vi "From Variant.vi"(8 "error in (no error)":errorcluster, 10 "Variant":variant, 11 "Abs_Double Float in":refnum<class "Abs_U32 Integer 1D.lvclass">) -> (0 "error out":errorcluster, 3 "Abs_Double Float out":refnum<class "Abs_U32 Integer 1D.lvclass">)   [LabVIEW 2021, in "Abs_U32 Integer 1D.lvclass"]
uses:
  Abs_U32 Integer 1D.lvclass
  Support/Type.ctl
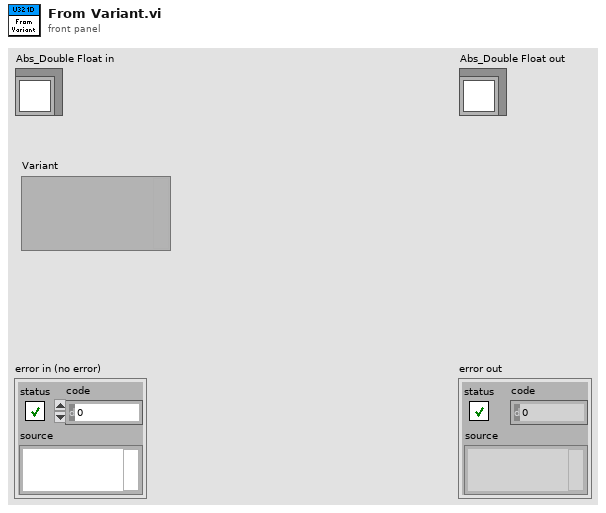
[diagram p1: front panel]
types:
  T1 = typedef "Abs_U32 Integer 1D.lvclass/Type.ctl" = u32[]
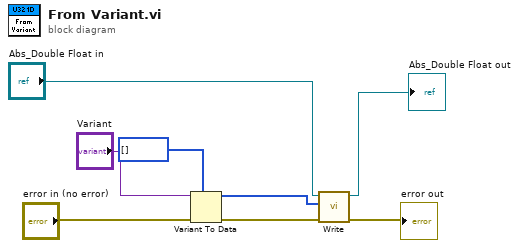
[diagram p0: block diagram]
diagram:
  n1 = Variant To Data(error in="error in (no error)", type=T1 [], Variant="Variant") -> (data=w7:T1, error out=w8:errorcluster)
  n2 = call-dynamic "Write.vi"("error in (no error)"=w8, "Value"=w7, "Double Float.lvclass in"="Abs_Double Float in") -> ("error out"=→"error out":errorcluster, "Double Float.lvclass out"=→"Abs_Double Float out":refnum<class "Abs_U32 Integer 1D.lvclass">)  [unwired: 7 in]
